vi "Get DDS Burst Period Ns.vi"(8 "error in (no error)":errorcluster, 11 "channel_index":u8) -> (0 "error out":errorcluster, 3 "function return":u32)   [LabVIEW 2021, in "vmmso.lvlib"]
doc: "DLL_API unsigned long long int WINAPI GetDDSBurstPeriodNs(unsigned char channel_index);"
uses:
  vmmso.lvlib
  vmmso.dll
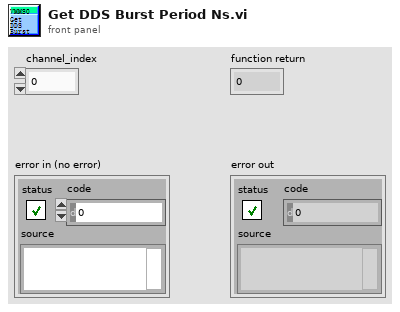
[diagram p1: front panel]
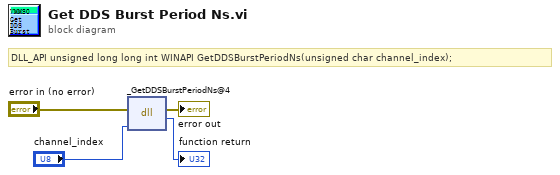
[diagram p0: block diagram]
diagram:
  # "DLL_API unsigned long long int WINAPI GetDDSBurstPeriodNs(unsigned char channel_index);"
  n1 = dll-call lib="O:/MSO/library/demo-Labview/vmmso/vmmso.*" fn="_GetDDSBurstPeriodNs@4"(error in="error in (no error)", "channel_index"="channel_index") -> (error out=→"error out":errorcluster, →"function return":u32)  [unwired: 3 in, 1 out]
